vi "ReMiRCVision.vi"() -> ()   [LabVIEW 2019]
uses:
  <vilib>/Analysis/coordinate.llb/2D Cartesian Coordinate Shift (Array).vi
  <vilib>/Analysis/coordinate.llb/2D Cartesian Coordinate Rotation (Array).vi
  <vilib>/vision/NI_Vision_Development_Module.lvlib
  <vilib>/Analysis/NI_AALPro.lvlib
  KNRm_ReMi_OS6_436Motor.lvlibp
panel:
  in  "RealWorldXY":cluster{"X":dbl, "Y":dbl}[][](array[cluster])=[[{"X"=-87.41918672815254, "Y"=-97.69950478545138}, {"X"=-44.676485154645185, "Y"=-97.86512942901233}, {"X"=1.0693055499785054, "Y"=-96.7577952889925}, {"X"=46.64075452454025, "Y"=-96.29119342235651}, {"X"=92.22082906177734, "Y"=-94.31936241201021}], [{"X"=-87.32274234871466, "Y"=-53.379030153432595}, {"X"=-43.46989684226859, "Y"=-51.8943192724522}, {"X"=0.9696666097077349, "Y"=-50.19260805869147}, {"X"=46.92217377535491, "Y"=-48.82417436459591}, {"X"=92.86040893315193, "Y"=-47.29622999450278}], [{"X"=-88.21280481186528, "Y"=-8.543006319347361}, {"X"=-42.795865235008016, "Y"=-7.3111011709588976}, {"X"=1.5816838876191233, "Y"=-6.615970435553383}, {"X"=47.03370209011219, "Y"=-4.021048175235278}, {"X"=93.9643907170363, "Y"=-1.4217991071066687}], [{"X"=-90.43482001089998, "Y"=35.789019295879484}, {"X"=-43.4846477445188, "Y"=38.11224916526762}, {"X"=2.3229241868558685, "Y"=39.03811614961179}, {"X"=46.863686527489115, "Y"=42.268175048978364}, {"X"=96.00471066315937, "Y"=43.92236372382627}], [{"X"=-93.42540075638188, "Y"=79.55955711607037}, {"X"=-44.09351543445324, "Y"=80.92850550222232}, {"X"=2.026996037323034, "Y"=84.04279899262731}, {"X"=49.043392430832846, "Y"=85.91841796569378}, {"X"=98.98878177149534, "Y"=89.88724663362977}]]
  out "element":dbl
  in  "DeltaXY":cluster{dbl, dbl}[][](array[cluster])=[[{-100.0, -100.0}, {-50.0, -100.0}, {0.0, -100.0}, {50.0, -100.0}, {100.0, -100.0}], [{-100.0, -50.0}, {-50.0, -50.0}, {0.0, -50.0}, {50.0, -50.0}, {100.0, -50.0}], [{-100.0, 0.0}, {-50.0, 0.0}, {0.0, 0.0}, {50.0, 0.0}, {100.0, 0.0}], [{-100.0, 50.0}, {-50.0, 50.0}, {0.0, 50.0}, {50.0, 50.0}, {100.0, 50.0}], [{-100.0, 100.0}, {-50.0, 100.0}, {0.0, 100.0}, {50.0, 100.0}, {100.0, 100.0}]]
  in  "vertical offset":cluster{"X":dbl, "Y":dbl}={"X"=2.0, "Y"=5.0} {"Y" format="%#_13g"; "X" format="%#_13g"}
  in  "horizontal offset":cluster{"X":dbl, "Y":dbl}={"X"=-4.0, "Y"=7.0} {"Y" format="%#_13g"; "X" format="%#_13g"}
  out "100%?":bool
  out "Boolean array":bool[](array[boolean])
  out "stop":bool
  out "botton":bool
  out "ColorDet Img":T1(plugin-control)
  out "G":u16
  out "B":u16
  out "Class":string
  out "output Brick (x, y, theta)":dbl[](array[numeric])
  in  "Grab":bool
  in  "Range (Threshold 1)":cluster{"Lower value":sgl, "Upper value":sgl}={"Lower value"=0.0, "Upper value"=110.0}
  out "Particle Measurements (Real-World)":dbl[][](array[numeric]) format="%.2f"
  in  "BCG Values (Brightness 1)":T2={"Brightness"=15.0, "Contrast"=82.15, "Gamma"=0.78999996}
  out "Number of Matches":i32
  out "Cal Img":T1(plugin-control)
  out "Bin Img":T1(plugin-control)
  in  "Stop Button":bool
  # "5"
  # "3"
  # "r"
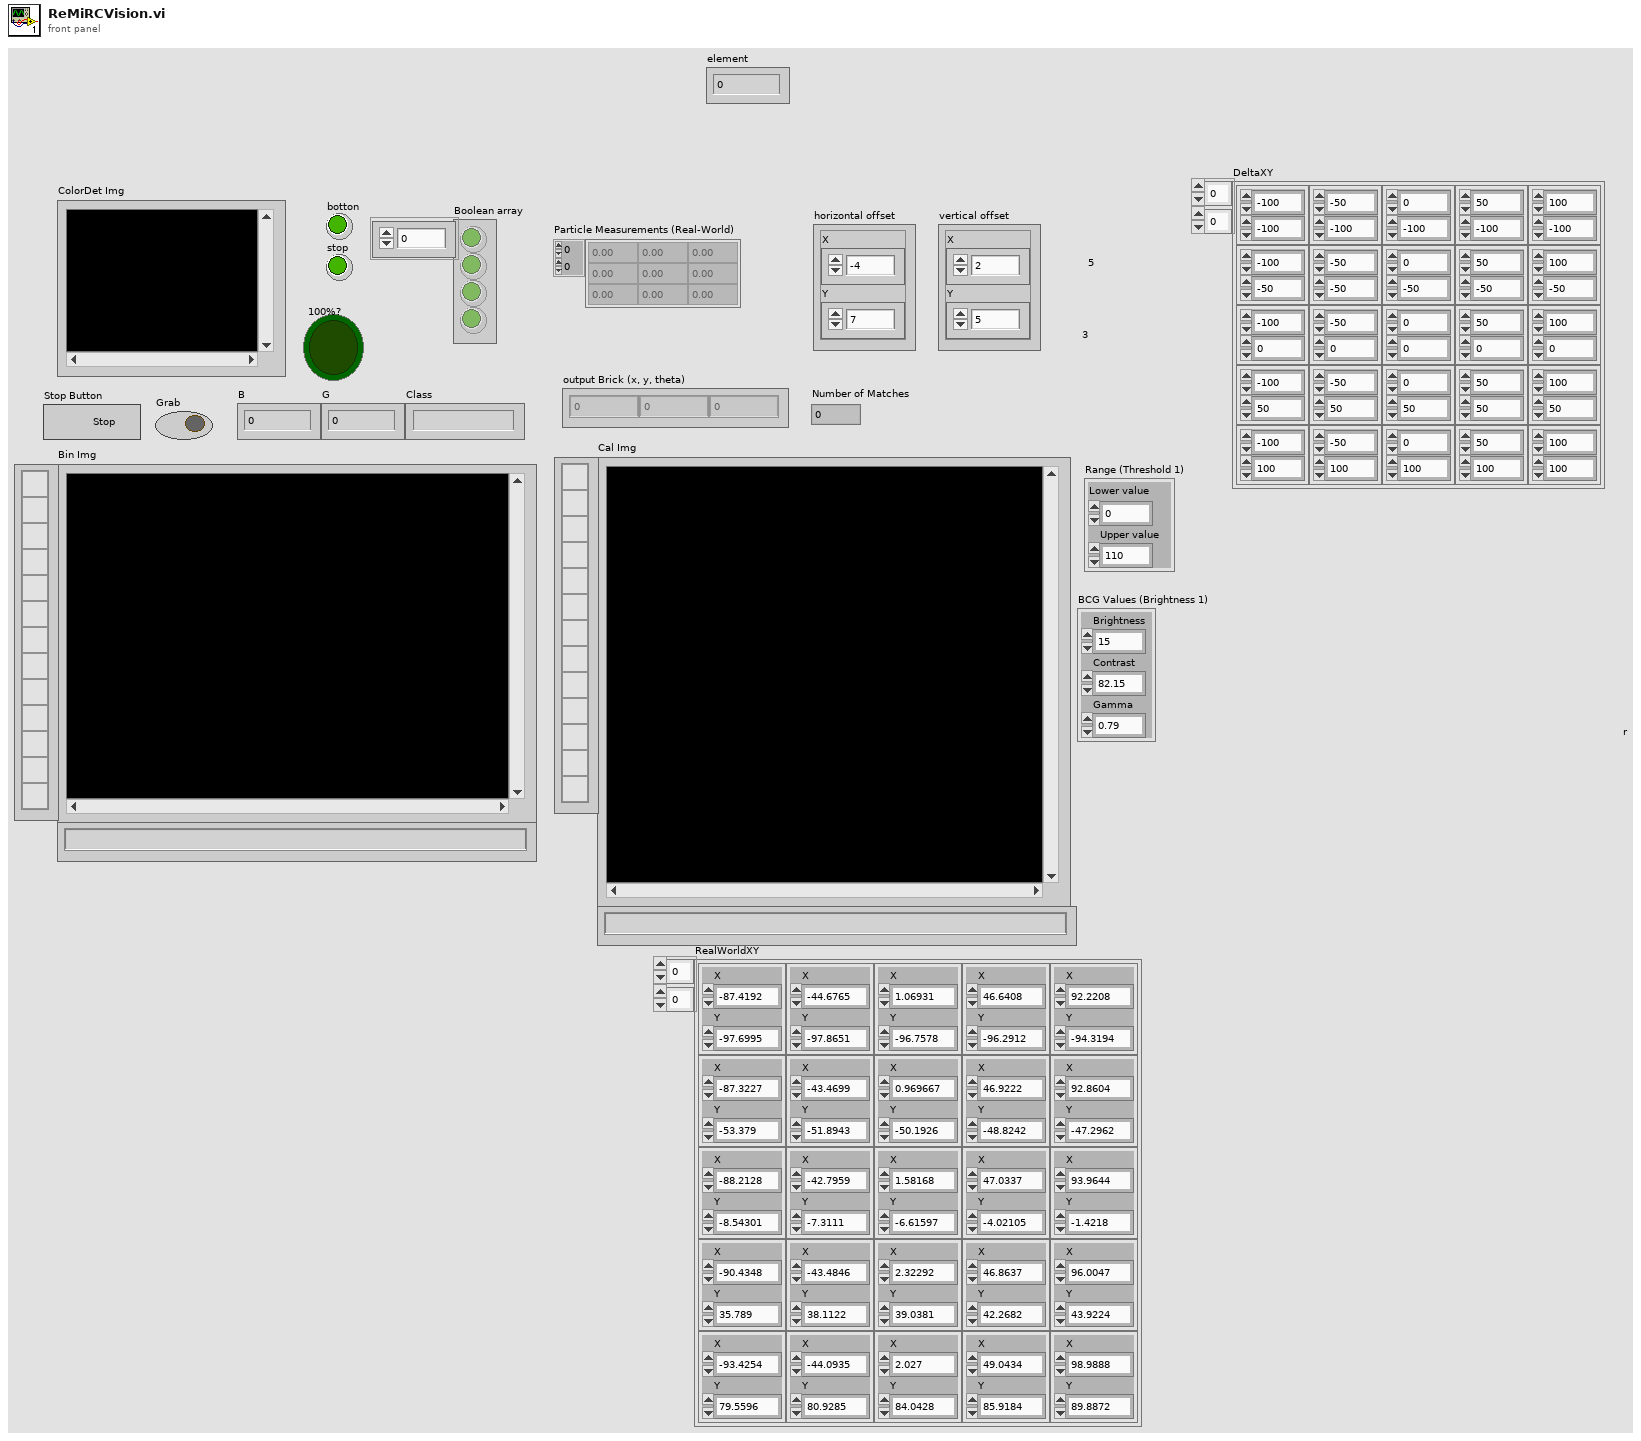
[diagram p1: front panel]
types:
  T1 = typedef "IMAQ Image.ctl" = refnum<image>
  T2 = cluster{"Brightness":sgl, "Contrast":sgl, "Gamma":sgl}
  T3 = typedef "Image Type" = u32
  T4 = cluster{"Interpolation Type":enum32{"Zero Order", "Bilinear", "Quadratic", "Cubic", "Bilinear Fixed"}, "Destination Width":u32, "Destination Height":u32, "Fill Value":sgl}
  T5 = cluster{"Particle Measurements (Real-World) (Particle Analysis 1)":dbl[], "Class":string}
  T6 = enum16{"P1", "P2", "P3", "P4", "P5", "P6", "OUT", "take a picture"}
  T7 = cluster{"Numeric":u8, "Numeric":u8, "Numeric":u8, "Numeric":u8}
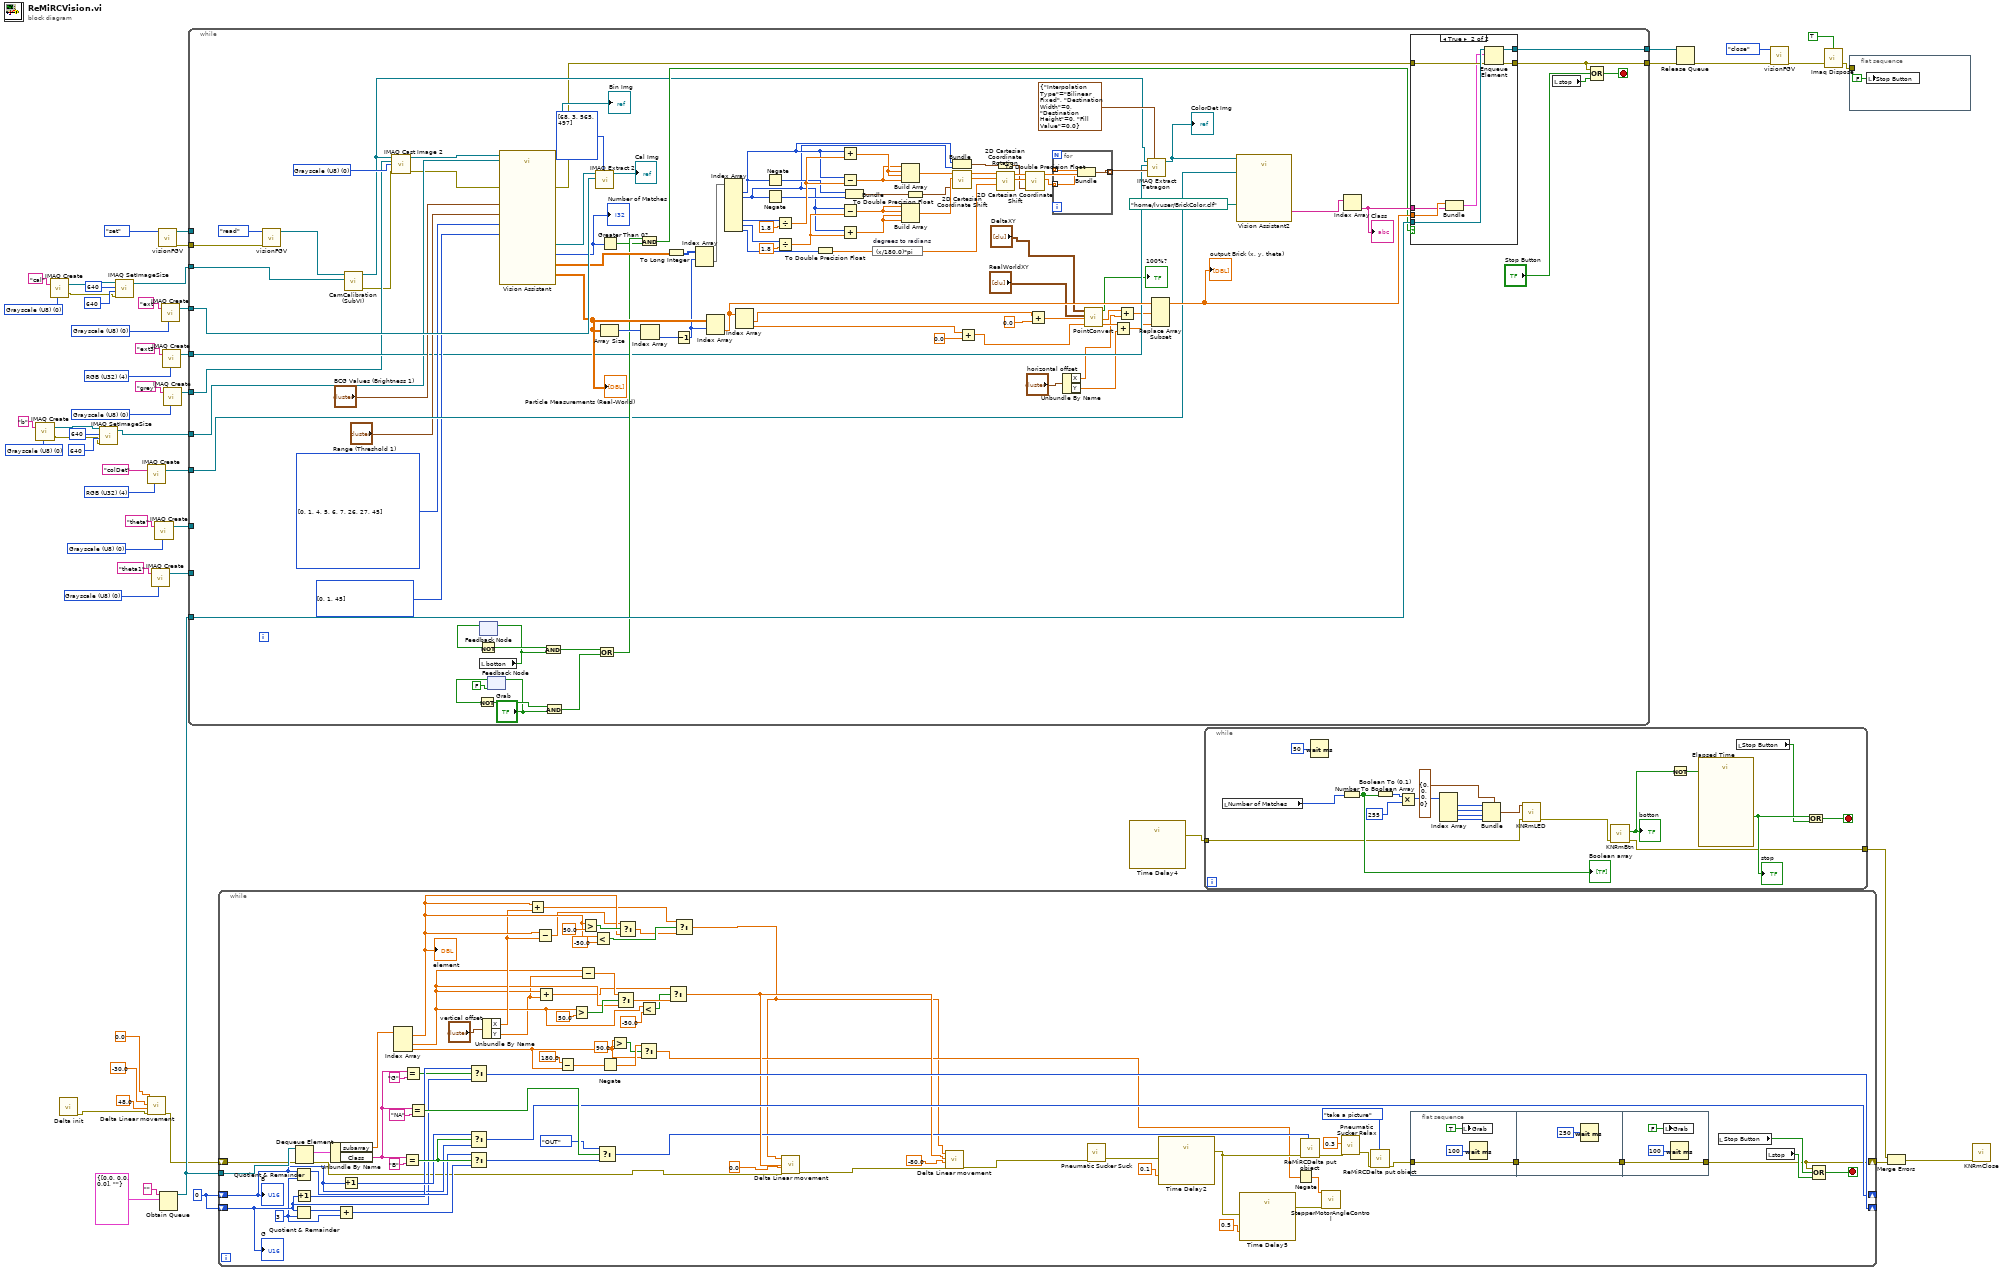
[diagram p0: block diagram]
diagram:
  w18 = T3 0 items=["Grayscale (U8)", "Grayscale (I16)", "Grayscale (SGL)", "Complex (CSG)", "RGB (U32)", "HSL (U32)", "RGB (U64)", "Grayscale (U16)"] ("Image Type")
  w23 = T3 0 items=["Grayscale (U8)", "Grayscale (I16)", "Grayscale (SGL)", "Complex (CSG)", "RGB (U32)", "HSL (U32)", "RGB (U64)", "Grayscale (U16)"] ("Image Type")
  w28 = T3 4 items=["Grayscale (U8)", "Grayscale (I16)", "Grayscale (SGL)", "Complex (CSG)", "RGB (U32)", "HSL (U32)", "RGB (U64)", "Grayscale (U16)"] ("Image Type")
  w30 = u16 0
  w33 = T3 4 items=["Grayscale (U8)", "Grayscale (I16)", "Grayscale (SGL)", "Complex (CSG)", "RGB (U32)", "HSL (U32)", "RGB (U64)", "Grayscale (U16)"] ("Image Type")
  w41 = T3 0 items=["Grayscale (U8)", "Grayscale (I16)", "Grayscale (SGL)", "Complex (CSG)", "RGB (U32)", "HSL (U32)", "RGB (U64)", "Grayscale (U16)"] ("Image Type")
  w44 = T3 0 items=["Grayscale (U8)", "Grayscale (I16)", "Grayscale (SGL)", "Complex (CSG)", "RGB (U32)", "HSL (U32)", "RGB (U64)", "Grayscale (U16)"] ("Image Type")
  w46 = T3 0 items=["Grayscale (U8)", "Grayscale (I16)", "Grayscale (SGL)", "Complex (CSG)", "RGB (U32)", "HSL (U32)", "RGB (U64)", "Grayscale (U16)"] ("Image Type")
  w48 = T3 0 items=["Grayscale (U8)", "Grayscale (I16)", "Grayscale (SGL)", "Complex (CSG)", "RGB (U32)", "HSL (U32)", "RGB (U64)", "Grayscale (U16)"] ("Image Type")
  n1 = call "IMAQ Create"("Image Name"="b", "Image Type"=w41) -> ("New Image"=w8:T1, "error out"=w7:errorcluster)  [unwired: 3 in]
  n2 = call "IMAQ Create"("Image Name"="cal", "Image Type"=w46) -> ("New Image"=w13:T1, "error out"=w12:errorcluster)  [unwired: 3 in]
  n3 = call "Delta init.vi"() -> ("error out"=w2:errorcluster)  [unwired: 9 in, 2 out]
  n4 = call "IMAQ SetImageSize"("error in (no error)"=w7, "Y Resolution"=640, "X Resolution"=640, "Image"=w8) -> ("Image Out"=w6:T1)  [unwired: 1 in, 1 out]
  n5 = call "IMAQ SetImageSize"("error in (no error)"=w12, "Y Resolution"=640, "X Resolution"=640, "Image"=w13) -> ("Image Out"=w11:T1)  [unwired: 1 in, 1 out]
  n6 = call "IMAQ Create"("Image Name"="colDet", "Image Type"=w33) -> ("New Image"=w32:T1)  [unwired: 3 in, 1 out]
  n7 = call "Delta Linear movement.vi"("error in (no error)"=w2, "z0"=48.0, "y0"=-30.0, "x0"=0.0) -> ("error out"=w1:errorcluster)  [unwired: 7 in]
  n8 = call "IMAQ Create"("Image Name"="theta1", "Image Type"=w18) -> ("New Image"=w17:T1)  [unwired: 3 in, 1 out]
  n9 = call "IMAQ Create"("Image Name"="theta", "Image Type"=w23) -> ("New Image"=w21:T1)  [unwired: 3 in, 1 out]
  n10 = call "visionFGV.vi"("Function"=enum16{"set", "read", "close"}."set") -> ("error out"=w50:errorcluster, "Image Out fgv"=w54:T1)  [unwired: 9 in]
  n11 = Obtain Queue(name (unnamed)="", element data type=cluster{"subarray":dbl[], "Class":string} {"subarray"=[0.0, 0.0, 0.0], "Class"=""}) -> (queue out=w38:refnum<queue>)  [unwired: 3 in, 2 out]
  n12 = call "IMAQ Create"("Image Name"="ext", "Image Type"=w44) -> ("New Image"=w43:T1)  [unwired: 3 in, 1 out]
  n13 = call "IMAQ Create"("Image Name"="ext3", "Image Type"=w28) -> ("New Image"=w27:T1)  [unwired: 3 in, 1 out]
  n14 = call "IMAQ Create"("Image Name"="grey", "Image Type"=w48) -> ("New Image"=w47:T1)  [unwired: 3 in, 1 out]
  n15 = while {
    tunnel: w54 -> [_]
    tunnel: w50 -> [w156]
    tunnel: w47 -> [w78]
    tunnel: w11 -> [w76]
    tunnel: w43 -> [w154]
    tunnel: w6 -> [w75]
    tunnel: w38 -> [w151]
    tunnel: [w101] -> w37
    tunnel: [w150] -> w35
    tunnel: w32 -> [w90]
    tunnel: w27 -> [w81]
    tunnel: w21 -> [_]
    tunnel: w17 -> [_]
    stop <- w98 stop-if-true
    w84 = i32[] [0, 1, 4, 5, 6, 7, 26, 27, 45] items=["Center of Mass X", "Center of Mass Y", "First Pixel X", "First Pixel Y", "Bounding Rect Left", "Bounding Rect Top", "Bounding Rect Right", "Bounding Rect Bottom", "Max Feret Diameter Start X", "Max Feret Diameter Start Y", "Max Feret Diameter End X", "Max Feret Diameter End Y", "Max Horiz. Segment Length Left", "Max Horiz. Segment Length Right", "Max Horiz. Segment Length Row", "-", "Bounding Rect Width", "Bounding Rect Height", "Bounding Rect Diagonal", "Perimeter", "Convex Hull Perimeter", "Holes' Perimeter", "Max Feret Diameter", "Equivalent Ellipse Major Axis", "Equivalent Ellipse Minor Axis", "Equivalent Ellipse Minor Axis (Feret)", "Equivalent Rect Long Side", "Equivalent Rect Short Side", "Equivalent Rect Diagonal", "Equivalent Rect Short Side (Feret)", "Average Horiz. Segment Length", "Average Vert. Segment Length", "Hydraulic Radius", "Waddel Disk Diameter", "-", "Area", "Holes' Area", "Particle & Holes' Area", "Convex Hull Area", "Image Area", "-", "Number of Holes", "Number of Horiz. Segments", "Number of Vert. Segments", "-", "Orientation", "Max Feret Diameter Orientation", "-", "% Area/Image Area", "% Area/(Particle & Holes' Area)", "Ratio of Equivalent Ellipse Axes", "Ratio of Equivalent Rect Sides", "-", "Elongation Factor", "Compactness Factor", "Heywood Circularity Factor", "Type Factor", "-", "Sum X", "Sum Y", "Sum XX", "Sum XY", "Sum YY", "Sum XXX", "Sum XXY", "Sum XYY", "Sum YYY", "-", "Moment of Inertia XX", "Moment of Inertia XY", "Moment of Inertia YY", "Moment of Inertia XXX", "Moment of Inertia XXY", "Moment of Inertia XYY", "Moment of Inertia YYY", "Norm. Moment of Inertia XX", "Norm. Moment of Inertia XY", "Norm. Moment of Inertia YY", "Norm. Moment of Inertia XXX", "Norm. Moment of Inertia XXY", "Norm. Moment of Inertia XYY", "Norm. Moment of Inertia YYY", "Hu Moment 1", "Hu Moment 2", "Hu Moment 3", "Hu Moment 4", "Hu Moment 5", "Hu Moment 6", "Hu Moment 7"] ("Pixel Measurements (Particle Analysis 1)")
    w83 = i32[] [0, 1, 45] items=["Center of Mass X", "Center of Mass Y", "First Pixel X", "First Pixel Y", "Bounding Rect Left", "Bounding Rect Top", "Bounding Rect Right", "Bounding Rect Bottom", "Max Feret Diameter Start X", "Max Feret Diameter Start Y", "Max Feret Diameter End X", "Max Feret Diameter End Y", "Max Horiz. Segment Length Left", "Max Horiz. Segment Length Right", "Max Horiz. Segment Length Row", "-", "Bounding Rect Width", "Bounding Rect Height", "Bounding Rect Diagonal", "Perimeter", "Convex Hull Perimeter", "Holes' Perimeter", "Max Feret Diameter", "Equivalent Ellipse Major Axis", "Equivalent Ellipse Minor Axis", "Equivalent Ellipse Minor Axis (Feret)", "Equivalent Rect Long Side", "Equivalent Rect Short Side", "Equivalent Rect Diagonal", "Equivalent Rect Short Side (Feret)", "Average Horiz. Segment Length", "Average Vert. Segment Length", "Hydraulic Radius", "Waddel Disk Diameter", "-", "Area", "Holes' Area", "Particle & Holes' Area", "Convex Hull Area", "Image Area", "-", "Number of Holes", "Number of Horiz. Segments", "Number of Vert. Segments", "-", "Orientation", "Max Feret Diameter Orientation", "-", "% Area/Image Area", "% Area/(Particle & Holes' Area)", "Ratio of Equivalent Ellipse Axes", "Ratio of Equivalent Rect Sides", "-", "Elongation Factor", "Compactness Factor", "Heywood Circularity Factor", "Type Factor", "-", "Sum X", "Sum Y", "Sum XX", "Sum XY", "Sum YY", "Sum XXX", "Sum XXY", "Sum XYY", "Sum YYY", "-", "Moment of Inertia XX", "Moment of Inertia XY", "Moment of Inertia YY", "Moment of Inertia XXX", "Moment of Inertia XXY", "Moment of Inertia XYY", "Moment of Inertia YYY", "Norm. Moment of Inertia XX", "Norm. Moment of Inertia XY", "Norm. Moment of Inertia YY", "Norm. Moment of Inertia XXX", "Norm. Moment of Inertia XXY", "Norm. Moment of Inertia XYY", "Norm. Moment of Inertia YYY", "Hu Moment 1", "Hu Moment 2", "Hu Moment 3", "Hu Moment 4", "Hu Moment 5", "Hu Moment 6", "Hu Moment 7"] ("Real-World Measurements (Particle Analysis 1)")
    w87 = T3 0 items=["Grayscale (U8)", "Grayscale (I16)", "Grayscale (SGL)", "Complex (CSG)", "RGB (U32)", "HSL (U32)", "RGB (U64)", "Grayscale (U16)"] ("Image Type")
    n16 = call "visionFGV.vi"("Error In"=w156, "Function"=enum16{"set", "read", "close"}."read") -> ("Image Out fgv"=w80:T1)  [unwired: 8 in, 1 out]
    n17 = call "CamCalibration (SubVI).vi"("Image Dst"=w76, "Image In"=w80) -> ("error out"=w73:errorcluster, "Image Out"=w77:T1)  [unwired: 8 in]
    n18 = call "IMAQ Cast Image 2"("Image Src"=w77, "Image Dst"=w78, "Image Type"=w87, "error in (no error)"=w73) -> ("Image Dst Out"=w69:T1, "error out"=w72:errorcluster)  [unwired: 10 in]
    n19 = feedback #1() -> (w96:bool)  [unwired: 1 in]
    n20 = Not(x=w96) -> (.not. x?=w95:bool)
    n21 = local read "botton"() -> (w94:bool)
    n22 = feedback-in #1(w94) -> ()
    n23 = feedback-in #2("Grab") -> ()
    n24 = feedback #2(FALSE ("Grab")) -> (w149:bool)
    n25 = Not(x=w149) -> (.not. x?=w148:bool)
    n26 = call "Vision Assistant"("Image In"=w69, "Image Dst"=w75, "BCG Values (Brightness 1)"="BCG Values (Brightness 1)", "Range (Threshold 1)"="Range (Threshold 1)", "Pixel Measurements (Particle Analysis 1)"=w84, "Real-World Measurements (Particle Analysis 1)"=w83, "error in"=w72) -> ("Image Out"=→"Bin Img":T1, "Number of Particles (Particle Analysis 1)"=w104:i32, "Particle Measurements (Real-World) (Particle Analysis 1)"=w145:dbl[][], "Particle Measurements (Pixels) (Particle Analysis 1)"=w140:dbl[][], "Image Buffer (Image Buffer 2)"=w143:T1, "error out"=w74:errorcluster)  [unwired: 15 in]
    "Number of Matches" <- w104
    "Particle Measurements (Real-World)" <- w145
    n27 = And(x=w95, y=w94) -> (x .and. y?=w93:bool)
    n28 = And(x=w148, y="Grab") -> (x .and. y?=w106:bool)
    n29 = call "IMAQ Extract 2"("Optional Rectangle"=i32[] [68, 3, 565, 497] ("Global Rectangle"), "Image Dst"=w154, "Image Src"=w143) -> ("Image Dst Out"=→"Cal Img":T1)  [unwired: 7 in, 1 out]
    n30 = Or(x=w93, y=w106) -> (x .or. y?=w105:bool)
    n31 = Array Size(array=w145) -> (size(s)=w146:i32[])
    n32 = Greater Than 0?(x=w104) -> (x > 0?=w103:bool)
    n33 = And(x=w105, y=w103) -> (x .and. y?=w102:bool)
    n34 = Index Array(array=w146) -> (element=w144:i32)  [unwired: 1 in]
    n35 = To Long Integer(number=w140) -> (32bit integer=w139:i32[][])
    n36 = Decrement(x=w144) -> (x-1=w82:i32)
    n37 = Index Array(array=w139, index (row)=w82) -> (element=w79:i32[])  [unwired: 1 in]
    n38 = Index Array(array=w145, index (row)=w82) -> (element=w142:dbl[])  [unwired: 1 in]
    n39 = Index Array(array=w79) -> (element #1=w120:i32, element #2=w119:i32, element #7=w130:i32, element #8=w126:i32, element #9=w133:i32)  [unwired: 9 in, 4 out]
    n40 = Index Array(array=w142) -> (element #1=w70:dbl, element #2=w71:dbl)  [unwired: 2 in]
    n41 = Negate(x=w120) -> (-x=w122:i32)
    n42 = Negate(x=w119) -> (-x=w123:i32)
    n43 = Divide(x=w130, y=1.8) -> (x/y=w128:dbl)
    n44 = Divide(x=w126, y=1.8) -> (x/y=w125:dbl)
    n45 = To Double Precision Float(number=w133) -> (double precision float=w124:dbl)
    n46 = Add(x=w120, y=w128) -> (x+y=w137:dbl)
    n47 = Subtract(x=w120, y=w128) -> (x-y=w136:dbl)
    n48 = Subtract(x=w119, y=w125) -> (x-y=w135:dbl)
    n49 = Add(x=w119, y=w125) -> (x+y=w134:dbl)
    n50 = Bundle(w122, w123) -> (w121:cluster{i32, i32})  [unwired: 1 in]
    n51 = expression code="(x/180.0)*pi" "degrees to radians"(w124) -> (w132:dbl)
    n52 = Build Array(w136, w137, w137, w136) -> (w118:dbl[])
    n53 = Build Array(w135, w135, w134, w134) -> (w117:dbl[])
    n54 = To Double Precision Float(number=w121) -> (double precision float=w108:cluster{dbl, dbl})
    n55 = Bundle("Numeric"=w120, "Numeric"=w119) -> (w112:cluster{"Numeric":i32, "Numeric":i32})  [unwired: 1 in]
    n56 = call-poly <vilib>:"2D Cartesian Coordinate Shift.vi"("shift"=w108, "Y"=w117, "X"=w118) -> ("Y Out"=w115:dbl[], "X Out"=w116:dbl[])  [unwired: 6 in, 1 out]
    n57 = Add(x=w71, y=0.0) -> (x+y=w58:dbl)
    n58 = To Double Precision Float(number=w112) -> (double precision float=w109:cluster{"Numeric":dbl, "Numeric":dbl})
    n59 = call-poly <vilib>:"2D Cartesian Coordinate Rotation.vi"("theta"=w132, "Y"=w115, "X"=w116) -> ("Y Out"=w113:dbl[], "X Out"=w114:dbl[])  [unwired: 6 in, 1 out]
    n60 = call-poly <vilib>:"2D Cartesian Coordinate Shift.vi"("shift"=w109, "Y"=w113, "X"=w114) -> ("Y Out"=w110:dbl[], "X Out"=w111:dbl[])  [unwired: 6 in, 1 out]
    n61 = Add(x=w70, y=0.0) -> (x+y=w67:dbl)
    n62 = for {
      tunnel: w111 -> [w160] mode=indexing
      tunnel: w110 -> [w159] mode=indexing
      tunnel: [w158] -> w131 mode=indexing
      n63 = Bundle("Numeric"=w160, "Numeric"=w159) -> (w158:cluster{"Numeric":dbl, "Numeric":dbl})  [unwired: 1 in]
    }
    n64 = Unbundle By Name("horizontal offset") -> ("X"=w60:dbl, "Y"=w59:dbl)
    n65 = call "PointConvert.vi"("RealWorldY"=w58, "RealWorldX"=w67, "RealWorldXY"="RealWorldXY", "DeltaXY"="DeltaXY") -> ("DeltaY"=w66:dbl, "DeltaX"=w64:dbl, "100%?"=→"100%?":bool)  [unwired: 5 in]
    n66 = Add(x=w66, y=w59) -> (x+y=w65:dbl)
    n67 = Add(x=w64, y=w60) -> (x+y=w63:dbl)
    n68 = call-poly "IMAQ Extract Tetragon"("Options"=T4 {"Interpolation Type"=enum."Bilinear Fixed", "Destination Width"=0, "Destination Height"=0, "Fill Value"=0.0}, "Tetragon"=w131, "Image Dst"=w81, "Image Src"=w77) -> ("Image Dst Out"=w91:T1)  [unwired: 6 in, 1 out]
    "ColorDet Img" <- w91
    n69 = Replace Array Subset(array=w142, new element #1=w63, new element #2=w65) -> (w141:dbl[])  [unwired: 2 in]
    "output Brick (x, y, theta)" <- w141
    n70 = call "Vision Assistant2"("Image In"=w91, "Image Dst"=w90, "File Path (Color Classification 1)"=path "/home/lvuser/BrickColor.clf") -> ("Classes (Color Classification 1)"=w89:string[])  [unwired: 22 in, 2 out]
    n71 = Index Array(array=w89) -> (element=w107:string)  [unwired: 1 in]
    "Class" <- w107
    n72 = case shown="True" w102 {
      tunnel: w151 -> [w161 w169]
      tunnel: w141 -> [_ w165]
      tunnel: [w162 w168] -> w101
      tunnel: w74 -> [w162 w167]
      tunnel: [w161 w166] -> w150
      tunnel: w107 -> [_ w164]
      frame False {
      }
      frame True {
        n73 = Bundle("Particle Measurements (Real-World) (Particle Analysis 1)"=w165, "Class"=w164) -> (w163:T5)  [unwired: 1 in]
        n74 = Enqueue Element(queue=w169, element=w163, error in (no error)=w167) -> (queue out=w166:refnum<queue>, error out=w168:errorcluster)  [unwired: 1 in, 1 out]
      }
    }
    n75 = local read "stop"() -> (w99:bool)
    n76 = Compound Arithmetic op=OR(w101, "Stop Button", w99) -> (w98:bool)
  }
  n77 = while {
    tunnel: w38 -> [w243]
    shift-right: [w208] -> w25
    shift-left: w1 -> [w242]
    shift-right: [w222] -> _
    shift-left: w30 -> [w221]
    shift-right: [w223] -> _
    shift-left: w30 -> [w220]
    stop <- w209 stop-if-true
    w218 = u16 3 ("y")
    n78 = Quotient & Remainder(x=w221, y=w218) -> (x-y*floor(x/y)=w228:u16)  [unwired: 1 out]
    n79 = Increment(x=w220) -> (x+1=w227:u16)
    n80 = Quotient & Remainder(x=w220, y=w218) -> (x-y*floor(x/y)=w219:u16)  [unwired: 1 out]
    n81 = Dequeue Element(queue=w243, error in (no error)=w242) -> (element=w236:cluster{"subarray":dbl[], "Class":string}, error out=w192:errorcluster)  [unwired: 1 in, 2 out]
    n82 = Unbundle By Name(w236) -> ("subarray"=w235:dbl[], "Class"=w225:string)
    n83 = Add(x=w219, y=w218) -> (x+y=w217:u16)
    n84 = Increment(x=w221) -> (x+1=w229:u16)
    n85 = Index Array(array=w235) -> (element #1=w182:dbl, element #2=w180:dbl, element #3=w189:dbl)  [unwired: 3 in]
    "element" <- w182
    n86 = Equal?(x=w225, y="B") -> (x = y?=w230:bool)
    n87 = Equal?(x=w225, y="G") -> (x = y?=w224:bool)
    n88 = Equal?(x=w225, y="NA") -> (x = y?=w233:bool)
    n89 = Select(t=w227, s=w224, f=w220) -> (s? t:f=w223:u16)
    n90 = Select(t=w229, s=w230, f=w221) -> (s? t:f=w222:u16)
    n91 = Select(t=w228, s=w230, f=w217) -> (s? t:f=w216:u16)
    n92 = Unbundle By Name("vertical offset") -> ("X"=w181:dbl, "Y"=w179:dbl)
    n93 = Add(x=w182, y=w181) -> (x+y=w177:dbl)
    n94 = Subtract(x=w182, y=w181) -> (x-y=w178:dbl)
    n95 = Add(x=w180, y=w179) -> (x+y=w175:dbl)
    n96 = Subtract(x=180.0, y=w189) -> (x-y=w238:dbl)
    n97 = Greater?(x=w180, y=50.0) -> (0:w213:bool)
    n98 = Subtract(x=w180, y=w179) -> (x-y=w176:dbl)
    n99 = Greater?(x=w182, y=50.0) -> (0:w186:bool)
    n100 = Less?(x=w182, y=-50.0) -> (x < y?=w185:bool)
    n101 = Select(t=T6."OUT" ("move to"), s=w233, f=w216) -> (s? t:f=w199:u16)
    n102 = Negate(x=w238) -> (-x=w237:dbl)
    n103 = Greater?(x=w189, y=90.0) -> (0:w215:bool)
    n104 = Select(t=w176, s=w213, f=w180) -> (s? t:f=w212:dbl)
    n105 = Select(t=w178, s=w186, f=w182) -> (s? t:f=w183:dbl)
    n106 = Less?(x=w180, y=-50.0) -> (x < y?=w204:bool)
    n107 = Select(t=w237, s=w215, f=w189) -> (s? t:f=w191:dbl)
    n108 = Select(t=w175, s=w204, f=w212) -> (s? t:f=w201:dbl)
    n109 = Select(t=w177, s=w185, f=w183) -> (s? t:f=w184:dbl)
    n110 = call "Delta Linear movement.vi"("error in (no error)"=w192, "z0"=0.0, "y0"=w201, "x0"=w184) -> ("error out"=w171:errorcluster)  [unwired: 7 in]
    n111 = call "Delta Linear movement.vi"("error in (no error)"=w171, "z0"=-80.0, "y0"=w201, "x0"=w184) -> ("error out"=w170:errorcluster)  [unwired: 7 in]
    n112 = call "Pneumatic Sucker Suck.vi"("error in"=w170) -> ("error out"=w196:errorcluster)  [unwired: 10 in]
    n113 = call "Time Delay2"("error in (no error)"=w196, "Delay Time (s)"=0.1) -> ("error out"=w194:errorcluster)  [unwired: 9 in]
    n114 = call "Time Delay5"("error in (no error)"=w194, "Delay Time (s)"=0.5) -> ("error out"=w193:errorcluster)  [unwired: 9 in]
    n115 = Negate(x=w191) -> (-x=w190:dbl)
    n116 = call "ReMiRCDelta put obiect.vi"("move to"=w199, "error in (no error)"=w194) -> ("error in (no error) 2"=w173:errorcluster)  [unwired: 9 in]
    n117 = call "StepperMotorAngleControl.vi"("error in"=w193, "angle"=w190) -> ()  [unwired: 9 in, 1 out]
    n118 = call "Pneumatic Sucker Relax.vi"("error in"=w173, "relax sec"=0.3) -> ("error out"=w172:errorcluster)  [unwired: 9 in]
    n119 = call "ReMiRCDelta put obiect.vi"("move to"=T6."take a picture", "error in (no error)"=w172) -> ("error in (no error) 2"=w198:errorcluster)  [unwired: 9 in]
    n120 = flat-sequence {
      tunnel: w198 -> [w246]
      tunnel: [w246] -> w206
      tunnel: [w247] -> w207
      tunnel: w206 -> [w247]
      tunnel: [w250] -> w208
      tunnel: w207 -> [w250]
      frame #0 {
        n121 = local write "Grab"(TRUE ("Grab")) -> ()
        n122 = Wait (ms)(milliseconds to wait=u32 100) -> ()  [unwired: 1 out]
      }
      frame #1 {
        n123 = Wait (ms)(milliseconds to wait=u32 250) -> ()  [unwired: 1 out]
      }
      frame #2 {
        n124 = local write "Grab"(FALSE ("Grab")) -> ()
        n125 = Wait (ms)(milliseconds to wait=u32 100) -> ()  [unwired: 1 out]
      }
    }
    n126 = local read "Stop Button"() -> (w211:bool)
    n127 = local read "stop"() -> (w210:bool)
    n128 = Compound Arithmetic op=OR(w208, w211, w210) -> (w209:bool)
    "B" <- w221
    "G" <- w220
  }
  n129 = call "Time Delay4"() -> ("error out"=w24:errorcluster)  [unwired: 11 in]
  n130 = while {
    tunnel: [w266] -> w26
    tunnel: w24 -> [w252]
    stop <- w269 stop-if-true
    n131 = local read "Number of Matches"() -> (w254:i32)
    n132 = Wait (ms)(milliseconds to wait=u32 50) -> ()  [unwired: 1 out]
    n133 = Number To Boolean Array(number=w254) -> (Boolean array=w253:bool[])
    "Boolean array" <- w253
    n134 = Boolean To (0,1)(Boolean=w253) -> (0, 1=w262:i16[])
    n135 = Multiply(x=w262, y=255) -> (x*y=w261:i32[])
    n136 = Index Array(array=w261) -> (element #1=w259:i32, element #2=w258:i32, element #3=w257:i32, element #4=w256:i32)  [unwired: 4 in]
    n137 = Bundle(cluster=T7 {"Numeric"=0, "Numeric"=0, "Numeric"=0, "Numeric"=0} ("LEDSet"), "Numeric"=w259, "Numeric"=w258, "Numeric"=w257, "Numeric"=w256) -> (w263:T7)
    n138 = call "KNRmLED.vi"("error in"=w252, "LEDSet"=w263) -> ("error out"=w255:errorcluster)  [unwired: 9 in]
    n139 = call "KNRmBtn.vi"("error in"=w255) -> ("error out"=w266:errorcluster, "myRIOButton"=w265:bool)  [unwired: 9 in]
    "botton" <- w265
    n140 = Not(x=w265) -> (.not. x?=w268:bool)
    n141 = call "Elapsed Time"("Reset"=w268) -> ("Time has Elapsed"=w271:bool)  [unwired: 11 in, 7 out]
    "stop" <- w271
    n142 = local read "Stop Button"() -> (w270:bool)
    n143 = Or(x=w271, y=w270) -> (x .or. y?=w269:bool)
  }
  n144 = Release Queue(queue=w35, error in (no error)=w37) -> (error out=w36:errorcluster)  [unwired: 1 in, 2 out]
  n145 = call "visionFGV.vi"("Error In"=w36, "Function"=enum16{"set", "read", "close"}."close") -> ("error out"=w51:errorcluster)  [unwired: 8 in, 1 out]
  n146 = call "Imaq Dispose"("All Images? (No)"=TRUE, "error in (no error)"=w51) -> ("error out"=w16:errorcluster)  [unwired: 4 in]
  n147 = flat-sequence {
    tunnel: w16 -> [_]
    frame #0 {
      n148 = local write "Stop Button"(FALSE ("Stop Button")) -> ()
    }
  }
  n149 = Merge Errors(w26, w25) -> (w20:errorcluster)
  n150 = call "KNRmClose.vi"("error in"=w20) -> ()  [unwired: 10 in, 1 out]
